vi "Condition VIs.vi"(6 "Conn Pane Terminals.Msg Output Indicator":i32[](array[numeric]), 8 "error in":errorcluster, 9 "Conn Pane Terminals.Msg Control":i32[](array[numeric]), 10 "VI Refs":T1) -> (0 "error out":errorcluster)   [LabVIEW 2025, in "_Msg Rescript.lvlib" / "_Msg Rescript.lvclass"]
uses:
  _Msg Rescript.lvclass
  _Msg Rescript.lvclass/_Msg Rescript.ctl
  VI Refs.ctl
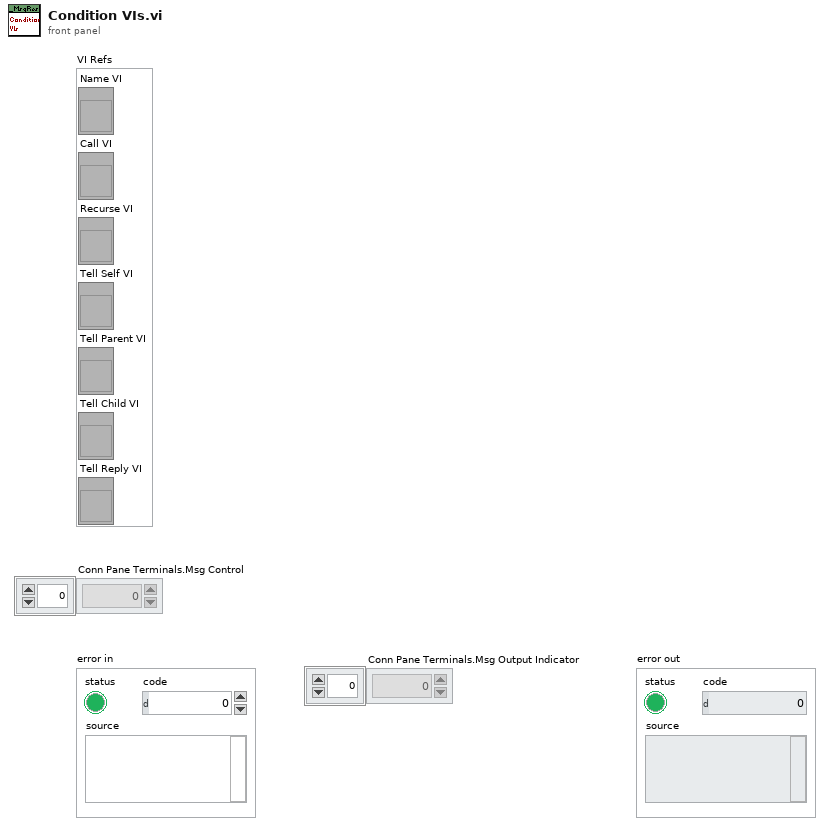
[diagram p1: front panel]
types:
  T1 = typedef "_Msg Rescript.lvlib/_Msg Rescript.lvclass/VI Refs.ctl" = cluster{"Name VI":refnum<vi>, "Call VI":refnum<vi>, "Recurse VI":refnum<vi>, "Tell Self VI":refnum<vi>, "Tell Parent VI":refnum<vi>, "Tell Child VI":refnum<vi>, "Tell Reply VI":refnum<vi>}
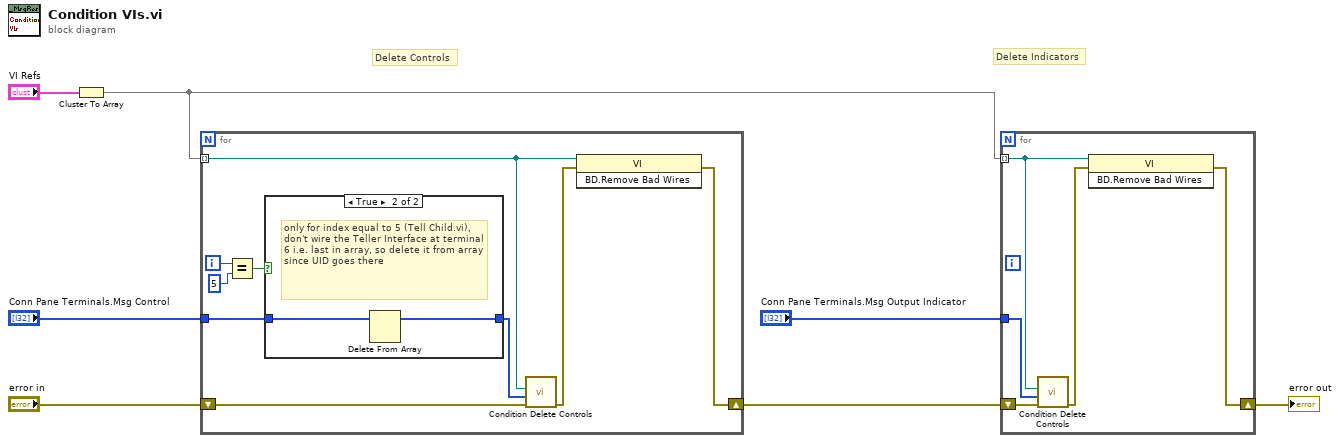
[diagram p0: block diagram]
diagram:
  # "Delete Indicators"
  # "Delete Controls"
  n1 = Cluster To Array(cluster="VI Refs") -> (array=w1:refnum<vi>[])
  n2 = for {
    tunnel: "Conn Pane Terminals.Msg Control" -> [w9]
    shift-right: [w14] -> w4
    shift-left: "error in" -> [w16]
    tunnel: w1 -> [w13] mode=indexing
    i -> [w10]
    n3 = Equal?(x=w10, y=5) -> (x = y?=w12:bool)
    n4 = case shown="True" w12 {
      tunnel: w9 -> [w17 w19]
      tunnel: [w17 w18] -> w8
      frame False {
      }
      frame True {
        # "only for index equal to 5 (Tell Child.vi), don't wire the Teller Interface at terminal 6 i.e. last in array, so delete it from array since UID goes there"
        n5 = Delete From Array(array=w19) -> (array with subset deleted=w18:i32[])  [unwired: 2 in, 1 out]
      }
    }
    n6 = call "Condition Delete Controls.vi"("error in"=w16, "Control Terminals"=w8, "VI Ref"=w13) -> ("error out"=w15:errorcluster)  [unwired: 8 in]
    n7 = invoke class="VI" method="BD.Remove Bad Wires"(reference=w13, error in=w15) -> (error out=w14:errorcluster)  [unwired: 1 in, 2 out]
  }
  n8 = for {
    tunnel: "Conn Pane Terminals.Msg Output Indicator" -> [w20]
    shift-right: [w22] -> w3
    shift-left: w4 -> [w24]
    tunnel: w1 -> [w21] mode=indexing
    n9 = call "Condition Delete Controls.vi"("error in"=w24, "Control Terminals"=w20, "VI Ref"=w21) -> ("error out"=w23:errorcluster)  [unwired: 8 in]
    n10 = invoke class="VI" method="BD.Remove Bad Wires"(reference=w21, error in=w23) -> (error out=w22:errorcluster)  [unwired: 1 in, 2 out]
  }
  "error out" <- w3
